vi "_Longlasting one-axis command.vi"(0 "System no.":i32=1 min=1 max=4 step=1, 2 "Axis to command":string="A", 3 "Command":string="ATZ", 4 "Value":dbl=nan format="%.6f", 5 "error in":errorcluster, 6 "Axis and value?":bool, 12 "Stop refnum":refnum<vi>) -> (14 "Answer":bool, 15 "Stopped":bool, 19 "error out":errorcluster)   [LabVIEW 2012]
doc: "This VI sends a command (like REF, MNL or MPL), polls with #7 for controller-ready signal and returns original (boolean) command response. \n\nValid for C-702, C-843, C-843.PM, C-844, C-848, C-865, C-866, C-880, C-880K005, E-710, E-761, F-206, Mercury™ (but must be present for E-517, E-712, E-725 and E-753 also)"
panel:
  in  "Local stop":bool
  # "This vi sends a command (like REF, MNL or MPL), \npolls with #7 for controller ready signal and\nreturns original (boolean) command response."
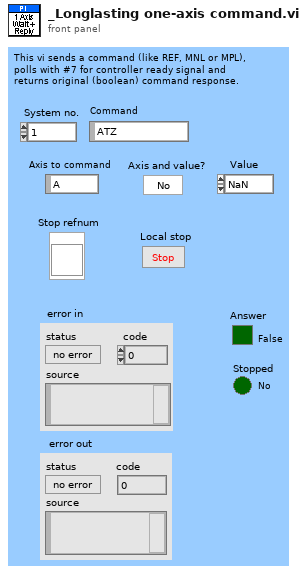
[diagram p1: front panel]
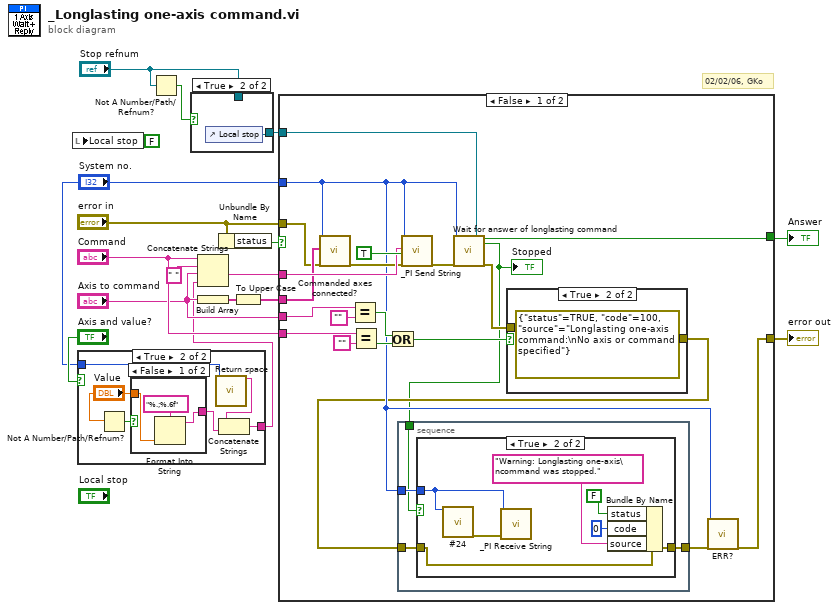
[diagram p0: block diagram]
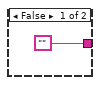
[diagram p3: hidden frame]
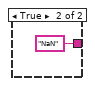
[diagram p4: hidden frame]
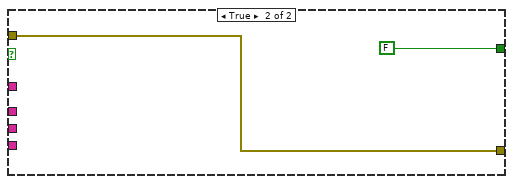
[diagram p7: hidden frame]
diagram:
  # "02/02/06, GKo"
  n1 = local write "Local stop"(FALSE ("Stop loop")) -> ()
  n2 = case shown="True" "Axis and value?" {
    tunnel: ["" w19] -> w7
    tunnel: "System no." -> [_ w21]
    frame False {
    }
    frame True {
      n3 = Not A Number/Path/Refnum?(number/path/refnum="Value") -> (NaN/Path/Refnum?=w23:bool)
      n4 = case shown="False" w23 {
        tunnel: "Value" -> [w26 _]
        tunnel: [w25 "NaN"] -> w22
        frame False {
          n5 = Format Into String(format string="%.;%.6f" ("Format String"), w26) -> (resulting string=w25:string)  [unwired: 2 in, 1 out]
        }
        frame True {
        }
      }
      n6 = call "Return space.vi"("System no."=w21) -> ("String out"=w20:string)  [unwired: 17 in, 1 out]
      n7 = Concatenate Strings(w20, w22) -> (w19:string)
    }
  }
  n8 = Not A Number/Path/Refnum?(number/path/refnum="Stop refnum") -> (NaN/Path/Refnum?=w4:bool)
  n9 = case shown="True" w4 {
    tunnel: [w29 w30] -> w2
    tunnel: "Stop refnum" -> [w29 _]
    frame False {
    }
    frame True {
      n10 = control-ref of="Local stop"() -> (w30:refnum<vi>)
    }
  }
  n11 = Concatenate Strings("Command", " ", "Axis to command", w7) -> (w17:string)
  n12 = Build Array("Axis to command") -> (w15:string[])
  n13 = Unbundle By Name("error in") -> ("status"=w11:bool)
  n14 = To Upper Case(1:w15) -> (0:w14:string[])
  n15 = case shown="False" w11 {
    tunnel: w17 -> [w50 _]
    tunnel: [w35 w67] -> w6
    tunnel: w14 -> [w48 _]
    tunnel: "System no." -> [w34 _]
    tunnel: "error in" -> [w47 w67]
    tunnel: "Axis to command" -> [w41 _]
    tunnel: "Command" -> [w40 _]
    tunnel: [w37 FALSE] -> w9
    tunnel: w2 -> [w33 _]
    frame False {
      n16 = call "Commanded axes connected?.vi"("System no."=w34, "Commanded axes"=w48, "error in"=w47) -> ("error out"=w49:errorcluster)  [unwired: 15 in, 1 out]
      n17 = Equal?(x=w41, y="" ("x")) -> (x = y?=w45:bool)
      n18 = Equal?(x=w40, y="" ("x")) -> (x = y?=w46:bool)
      n19 = Or(x=w45, y=w46) -> (x .or. y?=w42:bool)
      n20 = call "_PI Send String.vi"("System no."=w34, "String to send"=w50, "Attach termination char.?"=TRUE ("Attach Linefeed?"), "error in"=w49) -> ("error out"=w39:errorcluster)  [unwired: 15 in]
      n21 = call "Wait for answer of longlasting command.vi"("System no."=w34, "error in"=w39, "Stop refnum"=w33) -> ("Answer"=w37:bool, "Stopped"=w31:bool, "error out"=w38:errorcluster)  [unwired: 14 in]
      "Stopped" <- w31
      n22 = case shown="True" w42 {
        tunnel: [w64 errorcluster {"status"=TRUE, "code"=100, "source"="Longlasting one-axis command:\nNo axis or command specified"} ("error out")] -> w32
        tunnel: w38 -> [w64 _]
        frame False {
        }
        frame True {
        }
      }
      n23 = stacked-sequence {
        tunnel: w34 -> [w55]
        tunnel: w32 -> [w53]
        tunnel: w31 -> [w54]
        tunnel: [w52] -> w36
        frame #0 {
          n24 = case shown="True" w54 {
            tunnel: w55 -> [_ w63]
            tunnel: w53 -> [w56 w57]
            tunnel: [w56 w58] -> w52
            frame False {
            }
            frame True {
              n25 = call "#24.vi"("System no."=w63) -> ("error out"=w62:errorcluster)  [unwired: 18 in]
              n26 = call "_PI Receive String.vi"("System no."=w63, "error in"=w62) -> ()  [unwired: 15 in, 3 out]
              n27 = Bundle By Name(cluster=w57, "status"=FALSE, "code"=0, "source"="Warning: Longlasting one-axis\ncommand was stopped.") -> (w58:errorcluster)
            }
          }
        }
      }
      n28 = call "ERR?.vi"("System no."=w34, "error in"=w36) -> ("error out"=w35:errorcluster)  [unwired: 16 in, 1 out]
    }
    frame True {
    }
  }
  "error out" <- w6
  "Answer" <- w9
